vi "吸嘴偏移参数界面.vi"(8 "错误输入（无错误）":errorcluster, 10 "界面切换队列":refnum<queue>, 11 "VISA资源名称输入":refnum<visa-resource-name>) -> (0 "错误输出":errorcluster, 3 "VISA资源名称输出":refnum<visa-resource-name>)   [LabVIEW 2018]
panel:
  out "毫秒计时值":u32
  in  "枚举":T1(ring)
  in  "选项卡控件":enum32{"选项卡 1", "选项卡 2"}(tab)
  out "参数界面":bool
  out "烧录座位置补偿设定界面":bool
  out "手动界面":bool
  out "写R23+读R24+吸嘴2到光标位":bool
  out "写R21+读R22+吸嘴1到光标位":bool
  out "写R5D+读R5E+光标到光标位":bool
  out "写R172+读R172+吸嘴2设定":bool
  out "写R171+读R171+吸嘴1设定":bool
  out "写R170+读R170+光标设定":bool
  out "写DDT32560+Y轴吸嘴2":dbl
  out "写DDT32558+X轴吸嘴2":dbl
  out "写DDT32556+Y轴吸嘴1":dbl
  out "写DT32554+X轴吸嘴1":dbl
  out "写DDT32552+Y轴光标":dbl
  out "写DDT32550+X轴光标":dbl
  out "DDT90356":dbl
  out "DDT90348":dbl
  out "自动界面":bool
  out "手动界面":bool
  out "参数界面":bool
  out "IO界面":bool
  out "产品界面":bool
  out "字符串":string
  out "DDT90352":dbl
  out "DDT90360":dbl
  out "通讯周期":dbl
  out "DT1184":T2(ring)
  out "写R0+读R1+手动启动":bool
  out "写R8+读R9+机器复位":bool
  out "写R4+读R4+手动停止":bool
  # "X"
  # "Z1"
  # "Z2"
  # "Y"
  # "光标吸嘴参数"
  # "X轴"
  # "Y轴"
  # "光标"
  # "吸嘴1"
  # "吸嘴2"
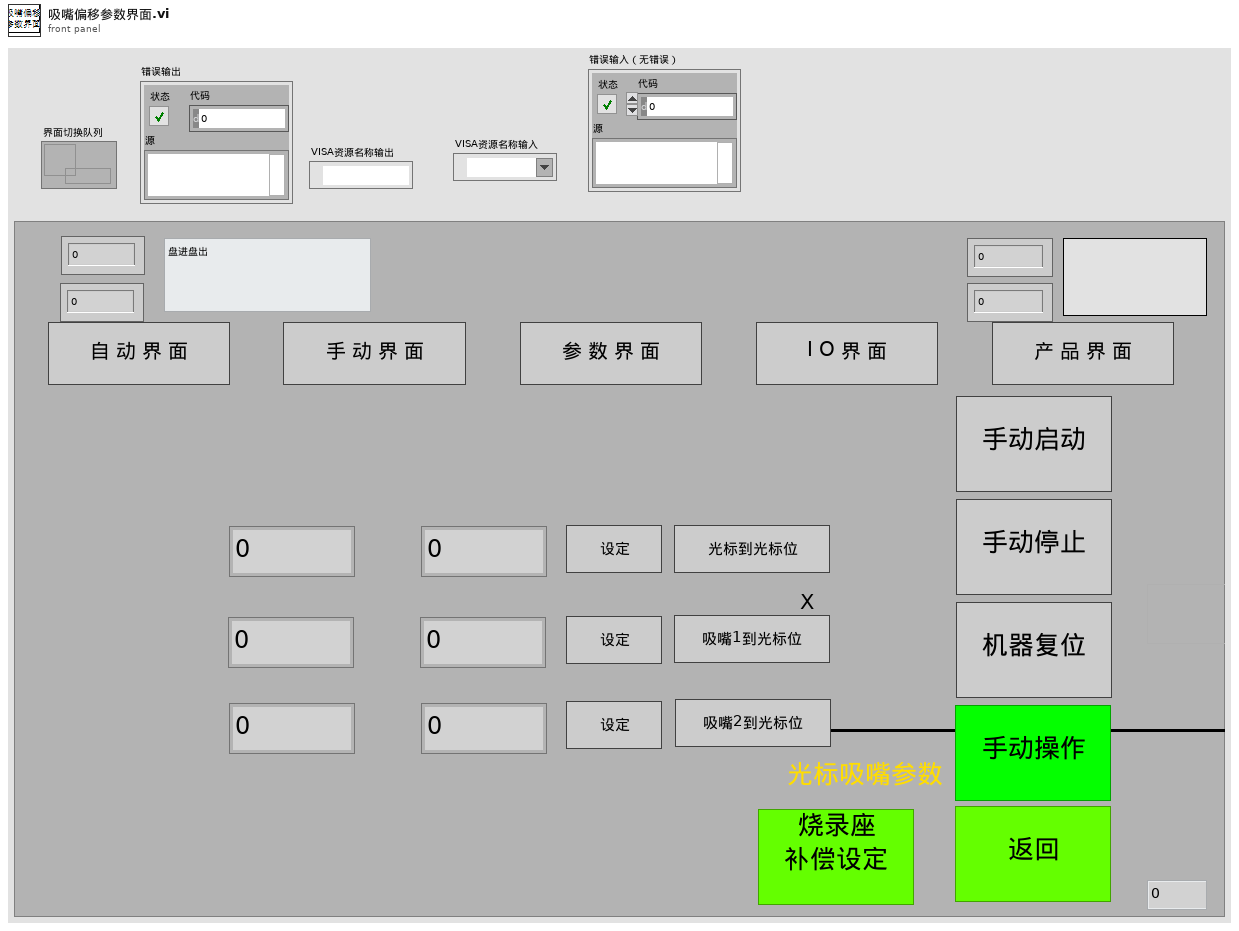
[diagram p1: front panel]
types:
  T1 = enum16{"读初始化", "读R170+8", "读R9+8", "读R5E+8", "读R1+8", "读R22+8位", "读DDT32560+5", "读DDT32550+5", "读DDT90356", "读DT1184", "读DDT90348", ""}
  T2 = enum16{"盘进盘出", "卷进卷出", "盘进卷出", "管进盘出", "管进卷出", "卷进盘出", ""}
  T3 = enum8{"Enabled", "Disabled", "Disabled and Grayed Out"}
  T4 = typedef "数据簇.ctl" = cluster{"字符串":string, "数值":i32, "布尔":bool}
  T5 = typedef "lveventtype.ctl" = enum32{"Null", "Timeout", "Annotation Menu Selection", "Annotation Menu Selection?", "App Instance Close", "App Instance Close?", "Autoscale Range Change", "Bookmark Info Change", "Cell Edit", "Cell Edit?", "Cursor Grab", "Cursor Grab?", "Cursor Menu Selection", "Cursor Menu Selection?", "Cursor Move", "Cursor Release", "Data Change", "Direction Change", "Display State Change", "Drag Ended", "Drag Enter", "Drag Leave", "Drag Over", "Drag Source Update", "Drag Starting", "Drag Starting?", "Drop", "Exec State Change", "Key Down", "Key Down?", "Key Repeat", "Key Repeat?", "Key Up", "Listbox Double Click", "Menu Activation?", "Menu Selection (App)", "Menu Selection? (App)", "Menu Selection (User)", "Mouse Down", "Mouse Down?", "Mouse Enter", "Mouse Leave", "Mouse Move", "Mouse Up", "Mouse Wheel", "NI Security User Change (App)", "Pane Size", "Panel Close", "Panel Close?", "Panel Resize", "Plot Attribute Change", "Scale Range Change", "Shortcut Menu Activation?", "Shortcut Menu Selection (App)", "Shortcut Menu Selection? (App)", "Shortcut Menu Selection (User)", "Tree Double Click", "Tree Drag", "Tree Drag?", "Tree Drop", "Tree Drop?", "Tree Item Close", "Tree Item Close?", "Tree Item Open", "Tree Item Open?", "User Event", "Value Change"}
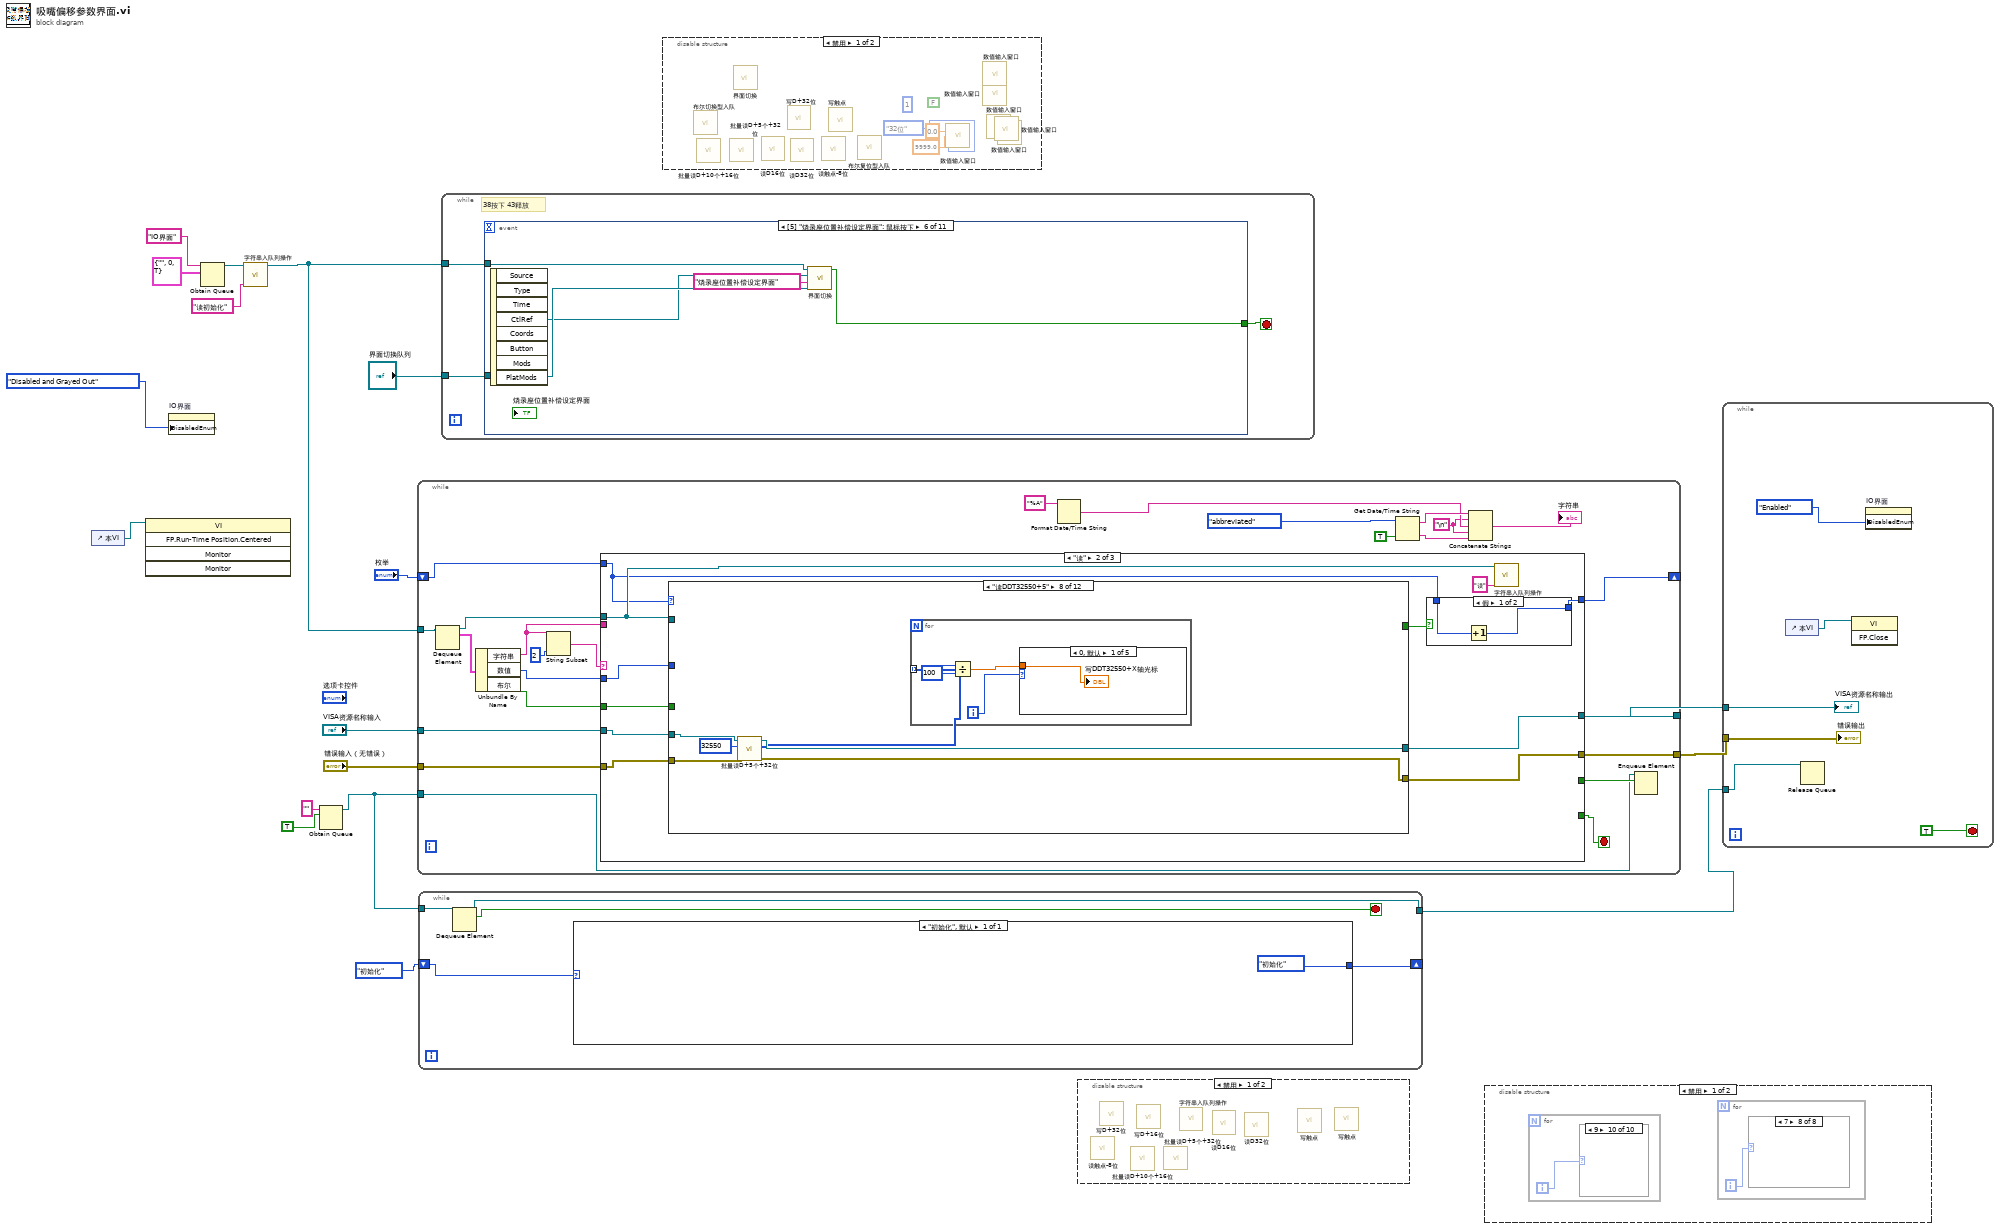
[diagram p0: block diagram]
diagram:
  n1 = control-ref of="本VI"() -> (w1:refnum<vi>)
  n2 = invoke class="VI" method="FP.Run-Time Position.Centered"(reference=w1) -> ()  [unwired: 4 in, 5 out]
  n3 = property on="IO界面" class="Bool"("DisabledEnum"=T3."Disabled and Grayed Out" ("禁用")) -> ()  [unwired: 2 in, 2 out]
  n4 = Obtain Queue(name (unnamed)="IO界面" ("名称（未命名）"), element data type=T4 {"字符串"="", "数值"=0, "布尔"=TRUE}) -> (queue out=w11:refnum<queue>)  [unwired: 3 in, 2 out]
  n5 = call "字符串入队列操作.vi"("字符消息入队列"="读初始化", "界面切换队列"=w11) -> ("队列输出"=w3:refnum<queue>)  [unwired: 9 in]
  n6 = Obtain Queue(name (unnamed)="" ("名称（未命名）"), element data type=TRUE) -> (queue out=w6:refnum<queue>)  [unwired: 3 in, 2 out]
  n7 = while {
    tunnel: w3 -> [w39]
    tunnel: "VISA资源名称输入" -> [w32]
    tunnel: "错误输入（无错误）" -> [w31]
    tunnel: [w30] -> w13
    tunnel: [w29] -> w12
    shift-right: [w26] -> _
    shift-left: "枚举" -> [w27]
    tunnel: w6 -> [w19]
    stop <- w21 stop-if-true
    w23 = "\n"
    n8 = Dequeue Element(queue=w39) -> (queue out=w36:refnum<queue>, element=w38:T4)  [unwired: 2 in, 2 out]
    n9 = Unbundle By Name(w38) -> ("字符串"=w33:string, "数值"=w35:i32, "布尔"=w34:bool)
    n10 = String Subset(string=w33, length (rest)=2 ("长度（剩余）")) -> (substring=w37:string)  [unwired: 1 in]
    n11 = case shown="\"读\"" w37 {
      selector: w37 -> [w46 _ _]
      tunnel: w36 -> [_ w54 w203]
      tunnel: w35 -> [_ w61 w202]
      tunnel: w34 -> [_ w60 w201]
      tunnel: w33 -> [_ _ w195]
      tunnel: w32 -> [w45 w59 w200]
      tunnel: w31 -> [w44 w58 w199]
      tunnel: [w45 w57 w197] -> w30
      tunnel: [w44 w56 w196] -> w29
      tunnel: [_ _ w198] -> w21
      tunnel: w27 -> [_ w52 _]
      tunnel: [_ w51 _] -> w26
      tunnel: [_ _ w193] -> w20
      frame "", Default {
        n12 = Concatenate Strings("无对应消息分支**" ("消息"), w46, "**" ("字符串"), "读写状态机" ("字符串")) -> (w48:string)
        n13 = One Button Dialog(message=w48) -> ()  [unwired: 1 in, 1 out]
      }
      frame "读" {
        n14 = case shown="\"读DDT32550+5\"" w52 {
          tunnel: w54 -> [_ _ _ _ _ _ _ _ _ _ _ _]
          tunnel: w61 -> [_ _ _ _ _ _ _ _ _ _ _ _]
          tunnel: w59 -> [w66 w73 w85 w95 w105 w116 w126 w137 w158 w167 w180 w192]
          tunnel: w58 -> [w65 w72 w84 w94 w104 w115 w125 w136 w157 w166 w179 w191]
          tunnel: [w66 w69 w81 w91 w101 w114 w124 w135 w156 w165 w178 w192] -> w57
          tunnel: [w65 w68 w80 w90 w100 w113 w123 w134 w155 w164 w177 w191] -> w56
          tunnel: w60 -> [_ _ _ _ _ _ _ _ _ _ _ _]
          tunnel: [_ _ _ _ _ _ _ _ _ _ _ TRUE] -> w53
          frame "读初始化" {
            n15 = Tick Count (ms)() -> (millisecond timer value=→"毫秒计时值":u32)
          }
          frame "读R170+8" {
            n16 = call "读触点-8位.vi"("error out"=w72, "触点类型"="R", "读取起始地址"="170", "VISA resource name out"=w73) -> ("error IO"=w68:errorcluster, "读取布尔数组"=w67:bool[], "VISA resource name out 2"=w69:refnum<visa-resource-name>)  [unwired: 4 in, 1 out]
            n17 = for {
              tunnel: w67 -> [w74] mode=indexing
              i -> [w75]
              n18 = case shown="2" w75 {
                tunnel: w74 -> [w76 w77 w78 _ _ _ _ _]
                frame 0, Default {
                  "写R170+读R170+光标设定" <- w76
                }
                frame 1 {
                  "写R171+读R171+吸嘴1设定" <- w77
                }
                frame 2 {
                  "写R172+读R172+吸嘴2设定" <- w78
                }
                frame 3 {
                }
                frame 4 {
                }
                frame 5 {
                }
                frame 6 {
                }
                frame 7 {
                }
              }
            }
          }
          frame "读R9+8" {
            n19 = call "读触点-8位.vi"("error out"=w84, "触点类型"="R", "读取起始地址"="9", "VISA resource name out"=w85) -> ("error IO"=w80:errorcluster, "读取布尔数组"=w79:bool[], "VISA resource name out 2"=w81:refnum<visa-resource-name>)  [unwired: 4 in, 1 out]
            n20 = for {
              tunnel: w79 -> [w86] mode=indexing
              i -> [w87]
              n21 = case shown="0, 默认" w87 {
                tunnel: w86 -> [w88 _ _ _ _ _ _ _]
                frame 0, Default {
                  "写R8+读R9+机器复位" <- w88
                }
                frame 1 {
                }
                frame 2 {
                }
                frame 3 {
                }
                frame 4 {
                }
                frame 5 {
                }
                frame 6 {
                }
                frame 7 {
                }
              }
            }
          }
          frame "读R5E+8" {
            n22 = call "读触点-8位.vi"("error out"=w94, "触点类型"="R", "读取起始地址"="5E", "VISA resource name out"=w95) -> ("error IO"=w90:errorcluster, "读取布尔数组"=w89:bool[], "VISA resource name out 2"=w91:refnum<visa-resource-name>)  [unwired: 4 in, 1 out]
            n23 = for {
              tunnel: w89 -> [w96] mode=indexing
              i -> [w97]
              n24 = case shown="0, 默认" w97 {
                tunnel: w96 -> [w98 _ _ _ _ _ _ _]
                frame 0, Default {
                  "写R5D+读R5E+光标到光标位" <- w98
                }
                frame 1 {
                }
                frame 2 {
                }
                frame 3 {
                }
                frame 4 {
                }
                frame 5 {
                }
                frame 6 {
                }
                frame 7 {
                }
              }
            }
          }
          frame "读R1+8" {
            n25 = call "读触点-8位.vi"("error out"=w104, "触点类型"="R", "读取起始地址"="1", "VISA resource name out"=w105) -> ("error IO"=w100:errorcluster, "读取布尔数组"=w99:bool[], "VISA resource name out 2"=w101:refnum<visa-resource-name>)  [unwired: 4 in, 1 out]
            n26 = for {
              tunnel: w99 -> [w106] mode=indexing
              i -> [w107]
              n27 = case shown="3" w107 {
                tunnel: w106 -> [w108 _ _ w109 _ _ _ _]
                frame 0, Default {
                  "写R0+读R1+手动启动" <- w108
                }
                frame 1 {
                }
                frame 2 {
                }
                frame 3 {
                  "写R4+读R4+手动停止" <- w109
                }
                frame 4 {
                }
                frame 5 {
                }
                frame 6 {
                }
                frame 7 {
                }
              }
            }
          }
          frame "读R22+8位" {
            n28 = call "读触点-8位.vi"("error out"=w115, "触点类型"="R", "读取起始地址"="22", "VISA resource name out"=w116) -> ("error IO"=w113:errorcluster, "读取布尔数组"=w112:bool[], "VISA resource name out 2"=w114:refnum<visa-resource-name>)  [unwired: 4 in, 1 out]
            n29 = for {
              tunnel: w112 -> [w117] mode=indexing
              i -> [w118]
              n30 = case shown="2" w118 {
                tunnel: w117 -> [w119 _ w120 _ _ _ _ _]
                frame 0, Default {
                  "写R21+读R22+吸嘴1到光标位" <- w119
                }
                frame 1 {
                }
                frame 2 {
                  "写R23+读R24+吸嘴2到光标位" <- w120
                }
                frame 3 {
                }
                frame 4 {
                }
                frame 5 {
                }
                frame 6 {
                }
                frame 7 {
                }
              }
            }
          }
          frame "读DDT32560+5" {
            n31 = call "批量读D+5个+32位.vi"("error out"=w125, "读取D地址"=32560, "VISA resource name out"=w126) -> ("error IO"=w123:errorcluster, "数组"=w122:i32[], "VISA resource name out 2"=w124:refnum<visa-resource-name>)  [unwired: 5 in, 1 out]
            n32 = for {
              tunnel: w122 -> [w127] mode=indexing
              i -> [w128]
              n33 = case shown="0, 默认" w128 {
                tunnel: w127 -> [w131 _ _ _ _]
                frame 0, Default {
                  n34 = Divide(x=w131, y=100) -> (x/y=→"写DDT32560+Y轴吸嘴2":dbl)
                }
                frame 1 {
                }
                frame 2 {
                }
                frame 3 {
                }
                frame 4 {
                }
              }
            }
          }
          frame "读DDT32550+5" {
            n35 = call "批量读D+5个+32位.vi"("error out"=w136, "读取D地址"=32550, "VISA resource name out"=w137) -> ("error IO"=w134:errorcluster, "数组"=w132:i32[], "VISA resource name out 2"=w135:refnum<visa-resource-name>)  [unwired: 5 in, 1 out]
            n36 = for {
              tunnel: w132 -> [w140] mode=indexing
              i -> [w141]
              n37 = Divide(x=w140, y=100) -> (x/y=w138:dbl)
              n38 = case shown="0, 默认" w141 {
                tunnel: w138 -> [w142 w143 w144 w145 w146]
                frame 0, Default {
                  "写DDT32550+X轴光标" <- w142
                }
                frame 1 {
                  "写DDT32552+Y轴光标" <- w143
                }
                frame 2 {
                  "写DT32554+X轴吸嘴1" <- w144
                }
                frame 3 {
                  "写DDT32556+Y轴吸嘴1" <- w145
                }
                frame 4 {
                  "写DDT32558+X轴吸嘴2" <- w146
                }
              }
            }
          }
          frame "读DDT90356" {
            n39 = call "批量读D+5个+32位.vi"("error out"=w157, "读取D地址"=90356, "VISA resource name out"=w158) -> ("error IO"=w155:errorcluster, "数组"=w161:i32[], "VISA resource name out 2"=w156:refnum<visa-resource-name>)  [unwired: 5 in, 1 out]
            n40 = Index Array(array=w161, index #1=0 ("索引"), index #2=2 ("索引")) -> (element #1=w154:i32, element #2=w153:i32)
            n41 = To Double Precision Float(number=w154) -> (double precision float=w152:dbl)
            n42 = To Double Precision Float(number=w153) -> (double precision float=w149:dbl)
            n43 = Divide(x=w152, y=100.0) -> (x/y=→"DDT90356":dbl)
            n44 = Divide(x=w149, y=100.0) -> (x/y=→"DDT90360":dbl)
          }
          frame "读DT1184" {
            n45 = call "读D16位.vi"("error out"=w166, "读取D地址"=1184, "VISA resource name out"=w167) -> ("error IO"=w164:errorcluster, "数值"=→"DT1184":u32, "VISA resource name out 2"=w165:refnum<visa-resource-name>)  [unwired: 5 in, 1 out]
          }
          frame "读DDT90348" {
            n46 = call "批量读D+5个+32位.vi"("error out"=w179, "读取D地址"=90348, "VISA resource name out"=w180) -> ("error IO"=w177:errorcluster, "数组"=w184:i32[], "VISA resource name out 2"=w178:refnum<visa-resource-name>)  [unwired: 5 in, 1 out]
            n47 = Index Array(array=w184, index #1=0 ("索引"), index #2=2 ("索引")) -> (element #1=w176:i32, element #2=w175:i32)
            n48 = To Double Precision Float(number=w175) -> (double precision float=w170:dbl)
            n49 = To Double Precision Float(number=w176) -> (double precision float=w174:dbl)
            n50 = Divide(x=w170, y=100.0) -> (x/y=→"DDT90352":dbl)
            n51 = Divide(x=w174, y=100.0) -> (x/y=→"DDT90348":dbl)
          }
          frame "" {
            n52 = local read "毫秒计时值"() -> (w188:u32)
            n53 = Tick Count (ms)() -> (millisecond timer value=w189:u32)
            n54 = Subtract(x=w189, y=w188) -> (x-y=w187:u32)
            n55 = Divide(x=w187, y=u32 1000) -> (x/y=→"通讯周期":dbl)
          }
        }
        n56 = case shown="假" w53 {
          tunnel: w52 -> [w63 _]
          tunnel: [w62 _] -> w51
          frame False {
            n57 = Increment(x=w63) -> (x+1=w62:T1)
          }
          frame True {
          }
        }
        n58 = call "字符串入队列操作.vi"("字符消息入队列"="读", "界面切换队列"=w54) -> ()  [unwired: 9 in, 1 out]
      }
      frame "写" {
        n59 = call "状态匹配.vi"("输入状态"=w195) -> ("输出状态"=w194:string)  [unwired: 10 in]
        n60 = case shown="\"写退出\"" w194 {
          selector: w194 -> [w206 _ _ _ _]
          tunnel: w203 -> [_ _ _ _ w246]
          tunnel: w202 -> [_ w212 w229 _ _]
          tunnel: w201 -> [_ _ _ w240 _]
          tunnel: w200 -> [w205 w222 w233 w245 w251]
          tunnel: w199 -> [w204 w221 w232 w244 w250]
          tunnel: [_ _ _ _ w249] -> w198
          tunnel: [w205 w220 w231 w243 w251] -> w197
          tunnel: [w204 w219 w230 w242 w250] -> w196
          tunnel: w195 -> [_ w211 w223 w234 _]
          tunnel: [_ _ _ _ w249] -> w193
          frame "", Default {
            n61 = Concatenate Strings("无对应消息分支**" ("消息"), w206, "**" ("字符串"), "写状态机" ("字符串")) -> (w210:string)
            n62 = One Button Dialog(message=w210) -> ()  [unwired: 1 in, 1 out]
          }
          frame "写DT" {
            n63 = String Length(string=w211) -> (length=w217:i32)
            n64 = Subtract(x=w217, y=4) -> (x-y=w215:i32)
            n65 = String Subset(string=w211, offset (0)=4 ("偏移量(0)"), length (rest)=w215) -> (substring=w214:string)
            n66 = Decimal String To Number(string=w214) -> (number=w213:i32)  [unwired: 2 in, 1 out]
            n67 = call "写D+16位.vi"("error out"=w221, "输入数值"=w212, "输入地址D"=w213, "VISA resource name out"=w222) -> ("error out 2"=w219:errorcluster, "VISA resource name out 2"=w220:refnum<visa-resource-name>)  [unwired: 3 in, 3 out]
          }
          frame "写DDT" {
            n68 = String Length(string=w223) -> (length=w227:i32)
            n69 = Subtract(x=w227, y=5) -> ()  [unwired: 1 out]
            n70 = String Subset(string=w223, offset (0)=5 ("偏移量(0)")) -> (substring=w224:string)  [unwired: 1 in]
            n71 = Decimal String To Number(string=w224) -> (number=w225:i32)  [unwired: 2 in, 1 out]
            n72 = call "写D+32位.vi"("error out"=w232, "输入数值"=w229, "输入地址D"=w225, "VISA resource name out"=w233) -> ("error out 2"=w230:errorcluster, "VISA resource name out 2"=w231:refnum<visa-resource-name>)  [unwired: 4 in, 2 out]
          }
          frame "写R" {
            n73 = String Length(string=w234) -> (length=w238:i32)
            n74 = Subtract(x=w238, y=3) -> (x-y=w236:i32)
            n75 = String Subset(string=w234, offset (0)=3 ("偏移量(0)"), length (rest)=w236) -> (substring=w235:string)
            n76 = call "写触点.vi"("布尔"=w240, "error out"=w244, "触点类型"="R", "写入起始地址"=w235, "VISA resource name out"=w245) -> ("error IO"=w242:errorcluster, "VISA resource name out 2"=w243:refnum<visa-resource-name>)  [unwired: 4 in, 1 out]
          }
          frame "写退出" {
            w249 = TRUE
            n77 = Flush Queue(queue=w246) -> (queue out=w247:refnum<queue>, error out=w248:errorcluster)  [unwired: 1 in, 1 out]
            n78 = Release Queue(queue=w247, error in (no error)=w248) -> ()  [unwired: 1 in, 3 out]
          }
        }
      }
    }
    n79 = Format Date/Time String(time format string (%c)="%A" ("时间格式字符串(%c)")) -> (date/time string=w24:string)  [unwired: 2 in]
    n80 = Get Date/Time String(date format (0)=enum16{"short", "long", "abbreviated"}."abbreviated" ("日期格式(0)"), want seconds? (F)=TRUE ("需要秒？(F)")) -> (date string=w41:string, time string=w22:string)  [unwired: 1 in]
    n81 = Concatenate Strings(w41, w23, w24, w23, w22) -> (→"字符串":string)
    n82 = Enqueue Element(queue=w19, element=w20) -> ()  [unwired: 2 in, 3 out]
  }
  n83 = while {
    shift-right: [w255] -> _
    shift-left: enum16{"初始化"}."初始化" -> [w256]
    tunnel: w6 -> [w254]
    tunnel: [w252] -> w5
    stop <- w253 stop-if-true
    n84 = Dequeue Element(queue=w254) -> (queue out=w252:refnum<queue>, element=w253:bool)  [unwired: 2 in, 2 out]
    n85 = case shown="\"初始化\", 默认" w256 {
      tunnel: [enum16{"初始化"}."初始化"] -> w255
      frame "初始化", Default {
      }
    }
  }
  n86 = while {
    tunnel: w3 -> [w259]
    tunnel: "界面切换队列" -> [w258]
    stop <- w260 stop-if-true
    # "38按下 43释放"
    n87 = event shown="[5] \"烧录座位置补偿设定界面\": 鼠标按下" {
      selector: _ -> [_ _ _ _ _ _ _ _ _ _ _]
      dyn-events: _ -> [_ _ _ _ _ _ _ _ _ _ _]
      timeout: _ -> [_ _ _ _ _ _ _ _ _ _ _]
      tunnel: [w264 w266 _ _ _ w311 w316 w321 w326 _ w333] -> w260
      tunnel: w259 -> [w265 w270 w273 w288 w289 w315 w320 w325 w330 _ w332]
      tunnel: w258 -> [w263 w269 _ _ _ w314 w319 w324 w329 _ w331]
      event "IO界面": Mouse Down {
        n88 = event-data() -> ("CtlRef"=w262:refnum<vi>)  [unwired: 1 in, 7 out]
        n89 = call "界面切换.vi"("界面切换队列输入"=w263, "切换界面名称输入"="IO界面", "Bool引用句柄"=w262, "状态转移输入"=w265) -> ("布尔"=w264:bool)  [unwired: 7 in]
      }
      event "参数界面", "参数界面": Mouse Down {
        n90 = event-data() -> ("CtlRef"=w268:refnum<vi>)  [unwired: 1 in, 7 out]
        n91 = call "界面切换.vi"("界面切换队列输入"=w269, "切换界面名称输入"="参数界面", "Bool引用句柄"=w268, "状态转移输入"=w270) -> ("布尔"=w266:bool)  [unwired: 7 in]
      }
      event "写R8+读R9+机器复位", "写R4+读R4+手动停止", "写R0+读R1+手动启动", "写R5D+读R5E+光标到光标位", "写R21+读R22+吸嘴1到光标位", "写R23+读R24+吸嘴2到光标位": Mouse Down; "写R8+读R9+机器复位", "写R4+读R4+手动停止", "写R0+读R1+手动启动", "写R5D+读R5E+光标到光标位", "写R21+读R22+吸嘴1到光标位", "写R23+读R24+吸嘴2到光标位": Mouse Up {
        n92 = event-data() -> ("Type"=w272:T5, "CtlRef"=w277:refnum<vi>)  [unwired: 1 in, 6 out]
        n93 = property class="Bool"(reference=w277) -> (reference out=w271:refnum<vi>, "Label.Text"=w276:string)  [unwired: 1 in, 1 out]
        n94 = Match Pattern(string=w276, regular expression="+" ("正则表达式")) -> (before substring=w274:string)  [unwired: 1 in, 3 out]
        n95 = call "布尔复位型入队.vi"("队列输入"=w273, "数值"=w272, "控件引用"=w271, "字符消息入队列"=w274) -> ()  [unwired: 2 in, 3 out]
      }
      event "写DDT32550+X轴光标", "写DDT32552+Y轴光标", "写DT32554+X轴吸嘴1", "写DDT32556+Y轴吸嘴1", "写DDT32558+X轴吸嘴2", "写DDT32560+Y轴吸嘴2": Mouse Down {
        n96 = event-data() -> ("CtlRef"=w287:refnum<vi>)  [unwired: 1 in, 7 out]
        n97 = property class="DigNum (严格)"(reference=w287) -> (reference out=w282:refnum<vi>, "Label.Text"=w286:string)  [unwired: 1 in, 1 out]
        n98 = Match Pattern(string=w286, regular expression="+" ("正则表达式")) -> (before substring=w284:string, after substring=w283:string)  [unwired: 1 in, 2 out]
        n99 = call "数值输入窗口.vi"("消息入队"=w288, "字符串"=w283, "字符消息入队列"=w284, "输入下限"=0.0, "输入上限"=99999999.0, "转换比例"=u32 100, "数据类型"=enum16{"32位", "16位"}."32位", "控件引用"=w282) -> ()  [unwired: 5 in, 3 out]
      }
      event "写R171+读R171+吸嘴1设定", "写R172+读R172+吸嘴2设定", "写R170+读R170+光标设定": Mouse Down {
        n100 = event-data() -> ("CtlRef"=w290:refnum<vi>)  [unwired: 1 in, 7 out]
        n101 = Two Button Dialog(message="确定设定？" ("消息")) -> (T button?=w291:bool)  [unwired: 2 in]
        n102 = case shown="真" w291 {
          tunnel: w290 -> [_ w304]
          tunnel: w289 -> [_ w306]
          frame False {
          }
          frame True {
            n103 = property class="Bool"(reference=w304) -> (reference out=w300:refnum<vi>, "Label.Text"=w303:string)  [unwired: 1 in, 1 out]
            n104 = Match Pattern(string=w303, regular expression="+" ("正则表达式")) -> (before substring=w301:string)  [unwired: 1 in, 3 out]
            n105 = call "布尔复位型入队.vi"("队列输入"=w306, "数值"=38, "控件引用"=w300, "字符消息入队列"=w301) -> ("队列输出"=w299:refnum<queue>, "控件引用 2"=w298:refnum<vi>, "字符消息出队列"=w297:string)  [unwired: 2 in]
            n106 = flat-sequence {
              tunnel: w299 -> [w308]
              tunnel: w298 -> [w309]
              tunnel: w297 -> [w310]
              tunnel: [w310] -> w296
              tunnel: [w309] -> w295
              tunnel: [w308] -> w294
              frame #0 {
                n107 = Wait (ms)(milliseconds to wait=u32 20 ("等待时间（毫秒）")) -> ()  [unwired: 1 out]
              }
            }
            n108 = call "布尔复位型入队.vi"("队列输入"=w294, "数值"=43, "控件引用"=w295, "字符消息入队列"=w296) -> ()  [unwired: 2 in, 3 out]
          }
        }
      }
      event "烧录座位置补偿设定界面": Mouse Down {
        n109 = event-data() -> ("CtlRef"=w313:refnum<vi>)  [unwired: 1 in, 7 out]
        n110 = call "界面切换.vi"("界面切换队列输入"=w314, "切换界面名称输入"="烧录座位置补偿设定界面", "Bool引用句柄"=w313, "状态转移输入"=w315) -> ("布尔"=w311:bool)  [unwired: 7 in]
      }
      event "产品界面": Mouse Down {
        n111 = event-data() -> ("CtlRef"=w318:refnum<vi>)  [unwired: 1 in, 7 out]
        n112 = call "界面切换.vi"("界面切换队列输入"=w319, "切换界面名称输入"="产品界面", "Bool引用句柄"=w318, "状态转移输入"=w320) -> ("布尔"=w316:bool)  [unwired: 7 in]
      }
      event "手动界面", "手动界面": Mouse Down {
        n113 = event-data() -> ("CtlRef"=w323:refnum<vi>)  [unwired: 1 in, 7 out]
        n114 = call "界面切换.vi"("界面切换队列输入"=w324, "切换界面名称输入"="手动界面", "Bool引用句柄"=w323, "状态转移输入"=w325) -> ("布尔"=w321:bool)  [unwired: 7 in]
      }
      event "自动界面": Mouse Down {
        n115 = event-data() -> ("CtlRef"=w328:refnum<vi>)  [unwired: 1 in, 7 out]
        n116 = call "界面切换.vi"("界面切换队列输入"=w329, "切换界面名称输入"="自动界面", "Bool引用句柄"=w328, "状态转移输入"=w330) -> ("布尔"=w326:bool)  [unwired: 7 in]
      }
      event Timeout {
        n117 = event-data() -> ()  [unwired: 1 in, 3 out]
      }
      event Panel Close? {
        n118 = event-data() -> ()  [unwired: 1 in, 4 out]
        n119 = Two Button Dialog(message="确定退出程序？" ("消息")) -> (T button?=w334:bool)  [unwired: 2 in]
        n120 = case shown="真" w334 {
          tunnel: [_ TRUE] -> w333
          tunnel: w332 -> [_ w339]
          tunnel: w331 -> [_ w338]
          frame False {
          }
          frame True {
            n121 = call "字符串入队列操作.vi"("字符消息入队列"="退出", "界面切换队列"=w338) -> ()  [unwired: 9 in, 1 out]
            n122 = call "字符串入队列操作.vi"("字符消息入队列"="写退出", "界面切换队列"=w339) -> ()  [unwired: 9 in, 1 out]
          }
        }
        n123 = event-data("Discard?"=TRUE ("放弃？")) -> ()  [unwired: 1 in, 1 out]
      }
    }
  }
  n124 = disable-structure shown="禁用" {
    frame Disabled {
      (unwired) u32 1 ("转换比例")
      (unwired) FALSE ("忽略数值上下限")
      n125 = call "布尔切换型入队.vi"() -> ()  [unwired: 12 in]
      n126 = call "批量读D+10个+16位.vi"() -> ()  [unwired: 8 in, 4 out]
      n127 = call "批量读D+5个+32位.vi"() -> ()  [unwired: 8 in, 4 out]
      n128 = call "界面切换.vi"() -> ()  [unwired: 11 in, 1 out]
      n129 = call "读D16位.vi"() -> ()  [unwired: 8 in, 4 out]
      n130 = call "写D+32位.vi"() -> ()  [unwired: 8 in, 4 out]
      n131 = call "读D32位.vi"() -> ()  [unwired: 9 in, 3 out]
      n132 = call "读触点-8位.vi"() -> ()  [unwired: 8 in, 4 out]
      n133 = call "写触点.vi"() -> ()  [unwired: 9 in, 3 out]
      n134 = call "布尔复位型入队.vi"() -> ()  [unwired: 6 in, 3 out]
      n135 = call "数值输入窗口.vi"("输入下限"=0.0, "输入上限"=9999.0, "数据类型"=enum16{"32位", "16位"}."32位") -> ("转换比例"=w345:u32)  [unwired: 9 in, 3 out]
      n136 = call "数值输入窗口.vi"() -> ()  [unwired: 13 in, 3 out]
      n137 = call "数值输入窗口.vi"() -> ()  [unwired: 13 in, 3 out]
      n138 = call "数值输入窗口.vi"() -> ()  [unwired: 13 in, 3 out]
      n139 = call "数值输入窗口.vi"() -> ()  [unwired: 13 in, 3 out]
      n140 = call "数值输入窗口.vi"() -> ()  [unwired: 13 in, 3 out]
    }
    frame Enabled {
    }
  }
  n141 = disable-structure shown="禁用" {
    frame Disabled {
      n142 = call "读触点-8位.vi"() -> ()  [unwired: 8 in, 4 out]
      n143 = call "写D+32位.vi"() -> ()  [unwired: 8 in, 4 out]
      n144 = call "批量读D+10个+16位.vi"() -> ()  [unwired: 8 in, 4 out]
      n145 = call "写D+16位.vi"() -> ()  [unwired: 7 in, 5 out]
      n146 = call "批量读D+5个+32位.vi"() -> ()  [unwired: 8 in, 4 out]
      n147 = call "字符串入队列操作.vi"() -> ()  [unwired: 11 in, 1 out]
      n148 = call "读D16位.vi"() -> ()  [unwired: 8 in, 4 out]
      n149 = call "读D32位.vi"() -> ()  [unwired: 9 in, 3 out]
      n150 = call "写触点.vi"() -> ()  [unwired: 9 in, 3 out]
      n151 = call "写触点.vi"() -> ()  [unwired: 9 in, 3 out]
    }
    frame Enabled {
    }
  }
  n152 = disable-structure shown="禁用" {
    frame Disabled {
      n153 = for {
        i -> [w347]
        n154 = case shown="9" w347 {
          frame 0, Default {
          }
          frame 1 {
          }
          frame 2 {
          }
          frame 3 {
          }
          frame 4 {
          }
          frame 5 {
          }
          frame 6 {
          }
          frame 7 {
          }
          frame 8 {
          }
          frame 9 {
          }
        }
      }
      n155 = for {
        i -> [w346]
        n156 = case shown="7" w346 {
          frame 0, Default {
          }
          frame 1 {
          }
          frame 2 {
          }
          frame 3 {
          }
          frame 4 {
          }
          frame 5 {
          }
          frame 6 {
          }
          frame 7 {
          }
        }
      }
    }
    frame Enabled {
    }
  }
  n157 = while {
    tunnel: w13 -> [w351]
    tunnel: w12 -> [w350]
    tunnel: w5 -> [w349]
    stop <- TRUE stop-if-true
    n158 = control-ref of="本VI"() -> (w352:refnum<vi>)
    n159 = Release Queue(queue=w349) -> ()  [unwired: 2 in, 3 out]
    n160 = invoke class="VI" method="FP.Close"(reference=w352) -> ()  [unwired: 2 in, 3 out]
    n161 = property on="IO界面" class="Bool"("DisabledEnum"=T3."Enabled" ("禁用")) -> ()  [unwired: 2 in, 2 out]
    "VISA资源名称输出" <- w351
    "错误输出" <- w350
  }
